vi "Finalize Inline Execution Units.vi"(8 "error in (no error)":errorcluster, 11 "RTStateVariables in":T1 {"Inline Execution Units"."Outgoing Data References"."Data Reference" format="%.0x"; "Inline Execution Units"."Incoming Data References" format="%.0x"}) -> (0 "error out":errorcluster, 3 "RTStateVariables out":T1 {"Inline Execution Units"."Outgoing Data References"."Data Reference" format="%.0x"; "Inline Execution Units"."Incoming Data References" format="%.0x"})   [LabVIEW 2020, in "Communication Bus Template Engine.lvlib"]
uses:
  Communication Bus Template Engine.lvlib
  Includes/Communication Bus Engine.lvlibp/Interfaces/Execution Unit/Execution Unit.lvclass
  <vilib>/NI/NIVS Inline Async API/_VS Inline Async API/VS Inline Async API/VS Inline Async API.lvclass
  RTStateVariables.ctl
  <vilib>/NI VeriStand/Custom Device API/Data Reference.ctl
  <vilib>/NI VeriStand/Custom Device API/Custom Device API.lvlib
  <vilib>/NI VeriStand/Custom Device API/Block Data Reference.ctl
  Inline Execution Unit Runtime Information.ctl
  Asynchronous Execution Unit Runtime Information.ctl
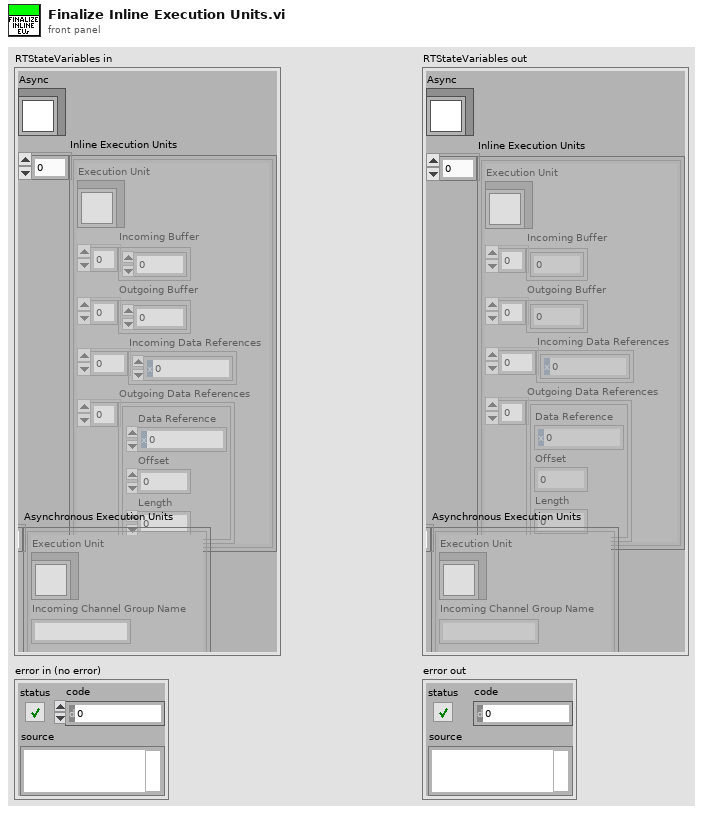
[diagram p1: front panel]
types:
  T1 = typedef "Communication Bus Template Engine.lvlib/RTStateVariables.ctl" = cluster{"Async":refnum<class "VS Inline Async API.lvclass">, "Inline Execution Units":T2[], "Asynchronous Execution Units":T5[]}
  T2 = typedef "Communication Bus Template Engine.lvlib/Inline Execution Unit Runtime Information.ctl" = cluster{"Execution Unit":refnum<class "Execution Unit.lvclass">, "Incoming Buffer":dbl[], "Outgoing Buffer":dbl[], "Incoming Data References":T3[], "Outgoing Data References":T4[]}
  T3 = typedef "Custom Device API.lvlib/Data Reference.ctl" = i32
  T4 = typedef "Custom Device API.lvlib/Block Data Reference.ctl" = cluster{"Data Reference":T3, "Offset":u64, "Length":u64}
  T5 = typedef "Communication Bus Template Engine.lvlib/Asynchronous Execution Unit Runtime Information.ctl" = cluster{"Execution Unit":refnum<class "Execution Unit.lvclass">, "Incoming Channel Group Name":string, "Outgoing Channel Group Name":string}
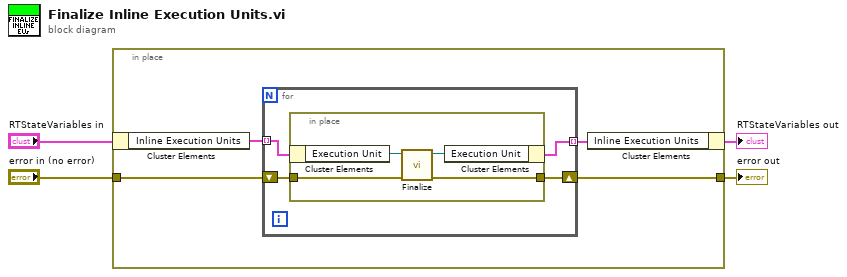
[diagram p0: block diagram]
diagram:
  n1 = in-place {
    in-place-border: [w8] -> w4
    in-place-border: "error in (no error)" -> [w7]
    n2 = in-place-cluster #1("RTStateVariables in") -> ("Inline Execution Units"=w6:T2[])
    n3 = for {
      shift-right: [w12] -> w8
      shift-left: w7 -> [w11]
      tunnel: w6 -> [w10] mode=indexing
      tunnel: [w9] -> w5 mode=indexing
      n4 = in-place {
        in-place-border: w11 -> [w14]
        in-place-border: [w13] -> w12
        n5 = in-place-cluster #2(w10) -> ("Execution Unit"=w16:refnum<class "Execution Unit.lvclass">)
        n6 = call-dynamic "Finalize.vi"("error in (no error)"=w14, "Execution Unit in"=w16) -> ("error out"=w13:errorcluster, "Execution Unit out"=w15:refnum<class "Execution Unit.lvclass">)  [unwired: 8 in]
        n7 = in-place-cluster #2("Execution Unit"=w15) -> (w9:T2)
      }
    }
    n8 = in-place-cluster #1("Inline Execution Units"=w5) -> (→"RTStateVariables out":T1)
  }
  "error out" <- w4
